vi "Call_enqueue.vi"(7 "Waveform":T6(array[cluster])=[{"first point time"=-0.004999939551282051, "xIncrement"=1e-07, "Waveforms"=array[100000 elements]}, {"first point time"=-0.004999939551282051, "xIncrement"=1e-07, "Waveforms"=array[100000 elements]}, {"first point time"=-0.004999939552429668, "xIncrement"=1e-07, "Waveforms"=array[100000 elements]}, {"first point time"=-0.004999939552429668, "xIncrement"=1e-07, "Waveforms"=array[100000 elements]}], 8 "error in":errorcluster, 10 "Input Data":T1 {"Estimate Source" items=["Any Source."=-2, "No Shot"=-1, "Basic Labview Estimate"=0, "IDL Estimate From Andrew"=1, "IDL Estimate From Keith"=2, "Old Metadata"=3]}, 11 "seconds since 1Jan1904":timestamp=timestamp(3428502400.8921742 s since 1904-01-01)) -> (0 "error IO":errorcluster)   [LabVIEW 2012]
uses:
  Private/Hardware ID.ctl
  Dust_Event.ctl
  Signal.ctl
  Private/Role ID.ctl
  Private/Estimate_source.ctl
panel:
  in  "First Detector\nHardware ID":T4=enum."CSA 2"
  in  "Second Detector\nHardware ID":T4=enum."CSA 3"
  in  "PSU Hardware ID":T4
  in  "Third Detector \nHardware ID":T4=enum."CSA 4"
  # "Dust Event"
  # "Signal"
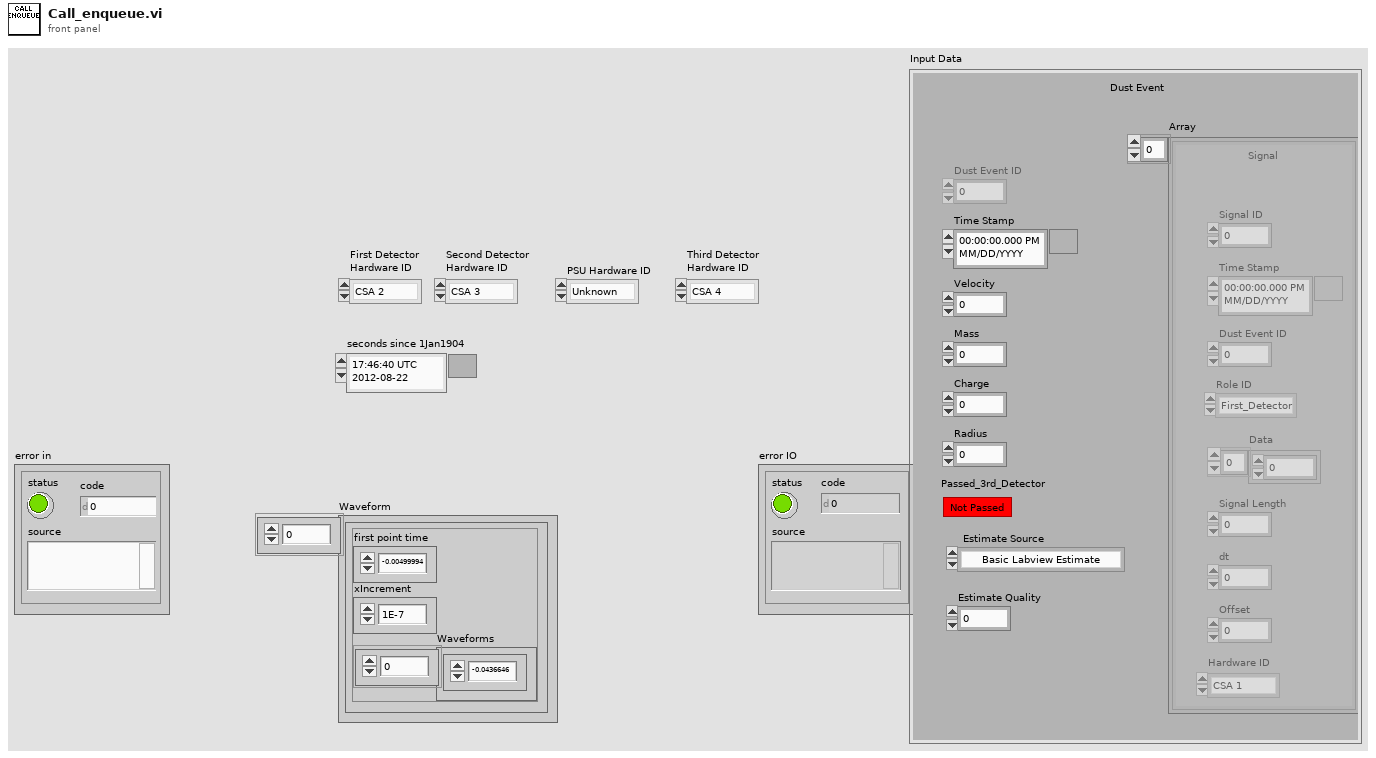
[diagram p1: front panel]
types:
  T1 = typedef "Dust_Event.ctl" = cluster{"Time Stamp":timestamp, "Velocity":sgl, "Mass":sgl, "Charge":sgl, "Radius":sgl, "Array":T2[], "Dust Event ID":i64, "Passed_3rd_Detector":bool, "Estimate Source":T5, "Estimate Quality":sgl}
  T2 = typedef "Signal.ctl" = cluster{"Signal ID":i64, "Time Stamp":timestamp, "Dust Event ID":i64, "Role ID":T3, "Data":sgl[], "Signal Length":i32, "dt":sgl, "Offset":dbl, "Hardware ID":T4}
  T3 = typedef "Role ID.ctl" = enum16{"First_Detector", "Second_Detector", "Third_Detector", "LeCroy_CH1", "LeCroy_CH2", "LeCroy_CH3", "LeCroy_CH4", "PSU"}
  T4 = typedef "Hardware ID.ctl" = enum16{"Unknown", "CSA 1", "CSA 2", "CSA 3", "CSA 4", "CSA 5", "CSA 6"}
  T5 = typedef "Estimate_source.ctl" = i8
  T6 = cluster{"first point time":dbl, "xIncrement":dbl, "Waveforms":dbl[]}[]
  T7 = enum16{"First_Detector", "Second_Detector", "Third_Detector", "LeCroy_CH1", "LeCroy_CH2", "LeCroy_CH3", "LeCroy_CH4"}
  T8 = cluster{"first point time":dbl, "xIncrement":dbl, "Waveforms":dbl[]}
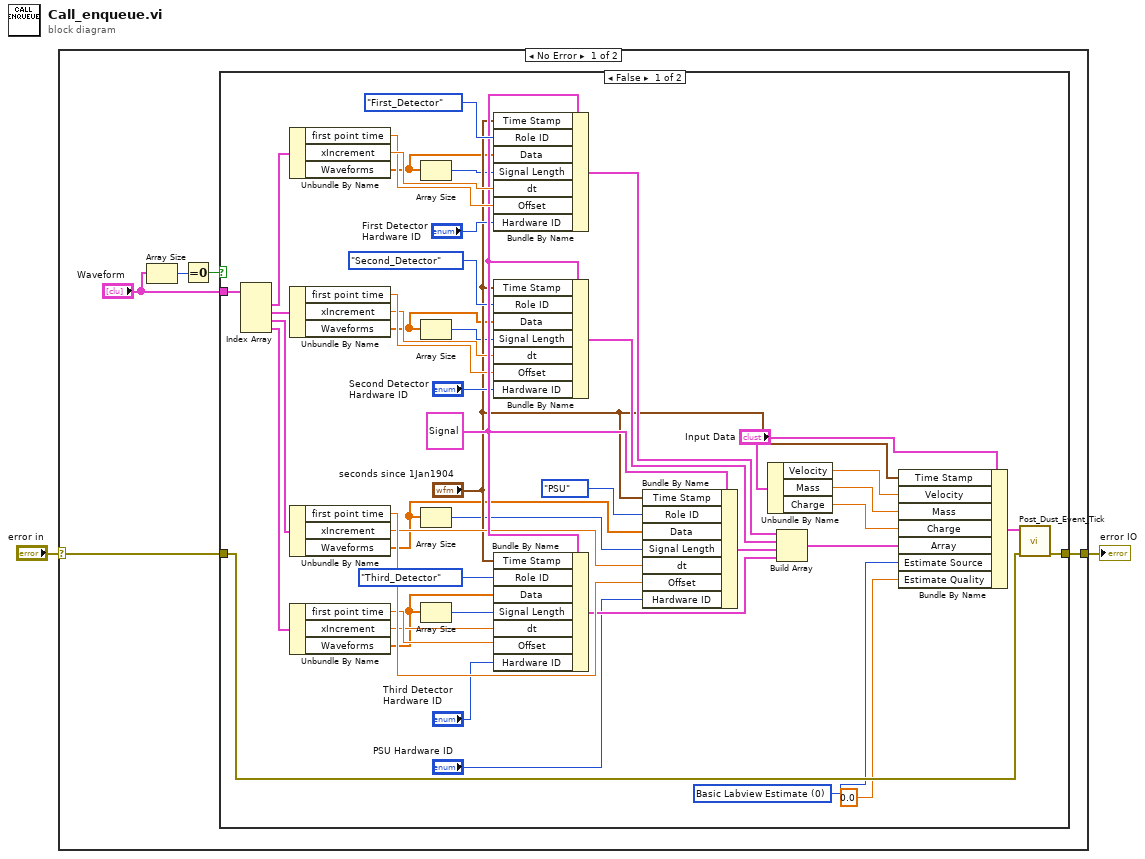
[diagram p0: block diagram]
diagram:
  n1 = case shown="No Error" "error in" {
    selector: "error in" -> [w4 w54]
    tunnel: [w7 w54] -> w1
    frame No Error {
      n2 = Array Size(array="Waveform") -> (size(s)=w6:i32)
      n3 = Equal To 0?(x=w6) -> (x = 0?=w5:bool)
      n4 = case shown="False" w5 {
        tunnel: "Waveform" -> [w51 _]
        tunnel: [w26 w53] -> w7
        tunnel: w4 -> [w25 w53]
        frame False {
          w21 = T5 0 items=["Basic Labview Estimate", "IDL Estimate"] ("Estimate Source")
          w44 = T2 {"Signal ID"=0, "Time Stamp"=timestamp(0 s since 1904-01-01), "Dust Event ID"=0, "Role ID"=enum."First_Detector", "Data"=[], "Signal Length"=0, "dt"=0.0, "Offset"=0.0, "Hardware ID"=enum."CSA 1"} ("Signal")
          n5 = Index Array(array=w51) -> (element #1=w50:T8, element #2=w33:T8, element #3=w46:T8, element #4=w45:T8)  [unwired: 4 in]
          n6 = Unbundle By Name(w50) -> ("first point time"=w48:dbl, "xIncrement"=w49:dbl, "Waveforms"=w11:dbl[])
          n7 = Unbundle By Name(w33) -> ("first point time"=w43:dbl, "xIncrement"=w42:dbl, "Waveforms"=w9:dbl[])
          n8 = Unbundle By Name(w46) -> ("first point time"=w37:dbl, "xIncrement"=w36:dbl, "Waveforms"=w13:dbl[])
          n9 = Unbundle By Name(w45) -> ("first point time"=w32:dbl, "xIncrement"=w31:dbl, "Waveforms"=w15:dbl[])
          n10 = Array Size(array=w11) -> (size(s)=w10:i32)
          n11 = Array Size(array=w9) -> (size(s)=w8:i32)
          n12 = Array Size(array=w13) -> (size(s)=w12:i32)
          n13 = Array Size(array=w15) -> (size(s)=w14:i32)
          n14 = Bundle By Name(cluster=w44, "Time Stamp"="seconds since 1Jan1904", "Role ID"=T7."First_Detector", "Data"=w11, "Signal Length"=w10, "dt"=w49, "Offset"=w48, "Hardware ID"="First Detector\nHardware ID") -> (w40:T2)
          n15 = Bundle By Name(cluster=w44, "Time Stamp"="seconds since 1Jan1904", "Role ID"=T7."Second_Detector", "Data"=w9, "Signal Length"=w8, "dt"=w42, "Offset"=w43, "Hardware ID"="Second Detector\nHardware ID") -> (w39:T2)
          n16 = Bundle By Name(cluster=w44, "Time Stamp"="seconds since 1Jan1904", "Role ID"=Role_ID."Third_Detector", "Data"=w15, "Signal Length"=w14, "dt"=w31, "Offset"=w32, "Hardware ID"="Third Detector \nHardware ID") -> (w30:T2)
          n17 = Bundle By Name(cluster=w44, "Time Stamp"="seconds since 1Jan1904", "Role ID"=Role_ID."PSU", "Data"=w13, "Signal Length"=w12, "dt"=w36, "Offset"=w37, "Hardware ID"="PSU Hardware ID") -> (w34:T2)
          n18 = Unbundle By Name("Input Data") -> ("Velocity"=w29:sgl, "Mass"=w28:sgl, "Charge"=w27:sgl)
          n19 = Build Array(w40, w39, w34, w30) -> (w38:T2[])
          n20 = Bundle By Name(cluster="Input Data", "Time Stamp"="seconds since 1Jan1904", "Velocity"=w29, "Mass"=w28, "Charge"=w27, "Array"=w38, "Estimate Source"=w21, "Estimate Quality"=sgl 0.0) -> (w52:T1)
          n21 = call "Post_Dust_Event_Tick.vi"("error in (no error)"=w25, "Input Data"=w52) -> ("error out"=w26:errorcluster)  [unwired: 8 in]
        }
        frame True {
        }
      }
    }
    frame Error {
    }
  }
  "error IO" <- w1
